vi "cw_3_6.vi"() -> ()   [LabVIEW 2022 SP3]
panel:
  in  "M":dbl
  out "Array 2":dbl[][](array[numeric])
  in  "Array":dbl[](array[numeric])
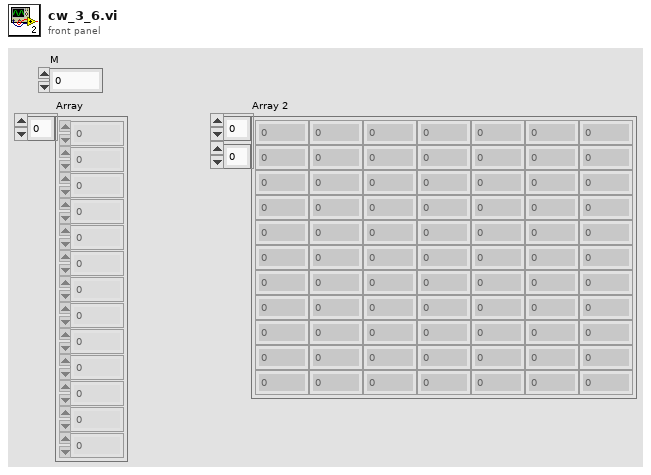
[diagram p1: front panel]
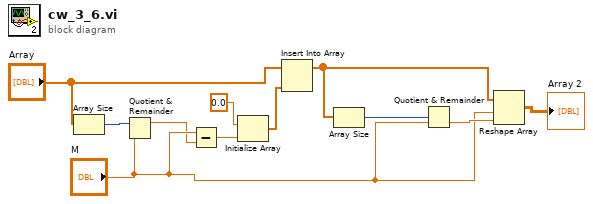
[diagram p0: block diagram]
diagram:
  n1 = Array Size(array="Array") -> (size(s)=w11:i32)
  n2 = Quotient & Remainder(x=w11, y="M") -> (x-y*floor(x/y)=w2:dbl)  [unwired: 1 out]
  n3 = Subtract(x="M", y=w2) -> (x-y=w1:dbl)
  n4 = Initialize Array(0.0 ("element"), w1) -> (w8:dbl[])
  n5 = Insert Into Array(array="Array", new element=w8) -> (w4:dbl[])  [unwired: 1 in]
  n6 = Array Size(array=w4) -> (size(s)=w7:i32)
  n7 = Quotient & Remainder(x=w7, y="M") -> (floor(x/y)=w5:dbl)  [unwired: 1 out]
  n8 = Reshape Array(w4, "M", w5) -> (→"Array 2":dbl[][])
